vi "Do.vi"(8 "error in (no error)":errorcluster, 10 "Numeric":dbl, 11 "object in":refnum<class "Base.lvclass">) -> (0 "error out":errorcluster, 2 "String":string, 3 "object out":refnum<class "Base.lvclass">)   [LabVIEW 2019, in "Base.lvclass"]
uses:
  Base.lvclass
  Base.lvclass/Base.ctl
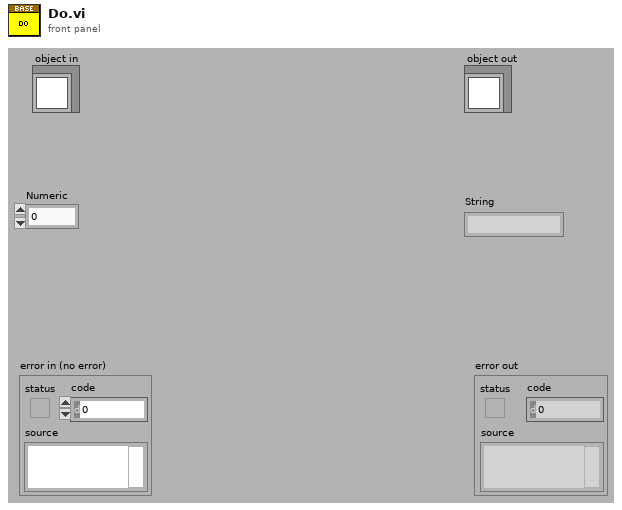
[diagram p1: front panel]
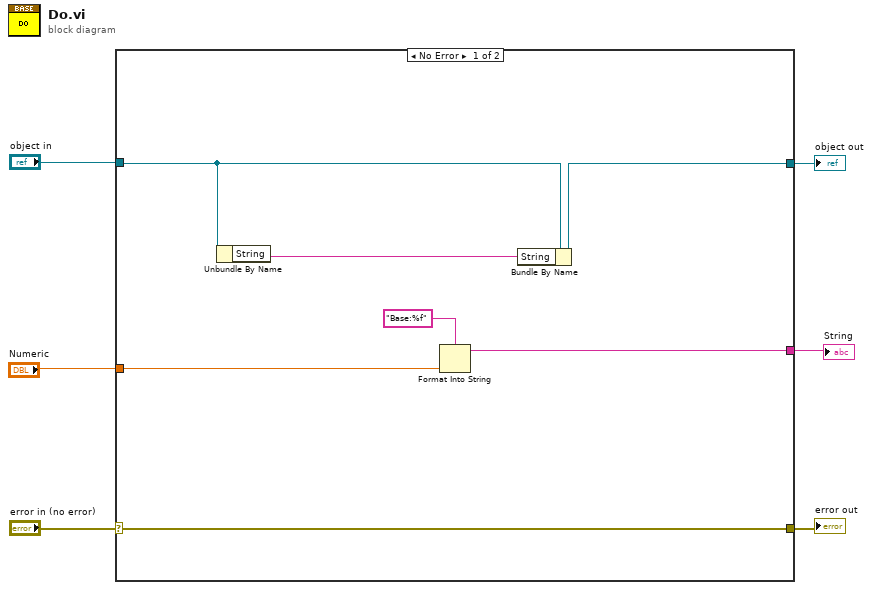
[diagram p0: block diagram]
diagram:
  n1 = case shown="No Error" "error in (no error)" {
    selector: "error in (no error)" -> [w12 w15]
    tunnel: [w12 w15] -> w5
    tunnel: [w10 w14] -> w3
    tunnel: "object in" -> [w11 w14]
    tunnel: "Numeric" -> [w8 _]
    tunnel: [w7 _] -> w1
    frame No Error {
      n2 = Unbundle By Name(w11) -> ("String"=w13:string)
      n3 = Format Into String(format string="Base:%f", w8) -> (resulting string=w7:string)  [unwired: 2 in, 1 out]
      n4 = Bundle By Name(cluster=w11, "String"=w13) -> (w10:refnum<class "Base.lvclass">)
    }
    frame Error {
    }
  }
  "error out" <- w5
  "object out" <- w3
  "String" <- w1
